vi "fpsCounter.vi"(8 "error in (no error)":errorcluster, 11 "Vision in":refnum<class "Vision.lvclass">) -> (0 "error out":errorcluster, 2 "Comm RX FPS":dbl, 3 "Vision out":refnum<class "Vision.lvclass">)   [LabVIEW 2018, in "Vision.lvclass"]
uses:
  Vision.lvclass
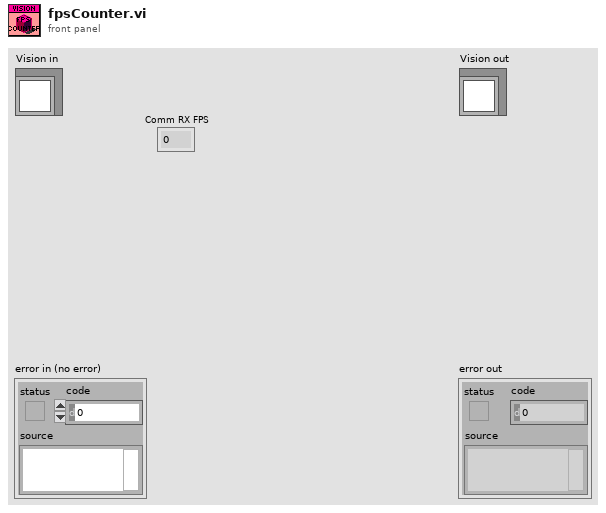
[diagram p1: front panel]
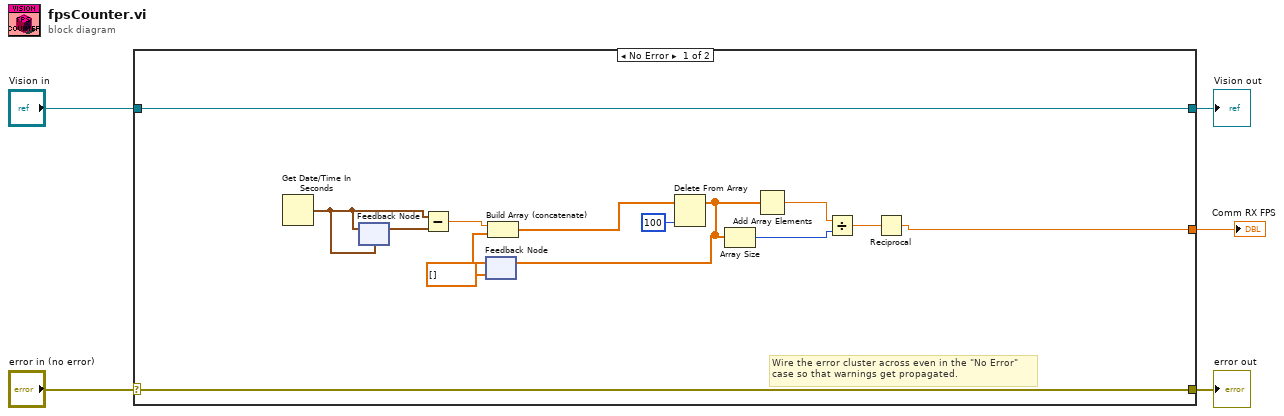
[diagram p0: block diagram]
diagram:
  n1 = case shown="No Error" "error in (no error)" {
    selector: "error in (no error)" -> [w18 w21]
    tunnel: [w18 w21] -> w4
    tunnel: [w19 w20] -> w2
    tunnel: "Vision in" -> [w19 w20]
    tunnel: [w6 _] -> w1
    frame No Error {
      # "Wire the error cluster across even in the \"No Error\"\ncase so that warnings get propagated."
      n2 = Get Date/Time In Seconds() -> (seconds since 1Jan1904=w7:timestamp)
      n3 = feedback #1(w7) -> (w8:timestamp)
      n4 = feedback-in #1(w7) -> ()
      n5 = Subtract(x=w7, y=w8) -> (x-y=w9:dbl)
      n6 = feedback #2(dbl[] []) -> (w10:dbl[])
      n7 = Build Array (concatenate)(w9, w10) -> (w12:dbl[])
      n8 = Delete From Array(array=w12, index=100) -> (array with subset deleted=w16:dbl[])  [unwired: 1 in, 1 out]
      n9 = feedback-in #2(w16) -> ()
      n10 = Array Size(array=w16) -> (size(s)=w15:i32)
      n11 = Add Array Elements(numeric array=w16) -> (sum=w14:dbl)
      n12 = Divide(x=w14, y=w15) -> (x/y=w17:dbl)
      n13 = Reciprocal(x=w17) -> (1/x=w6:dbl)
    }
    frame Error {
    }
  }
  "error out" <- w4
  "Vision out" <- w2
  "Comm RX FPS" <- w1
